vi "Is Set.vi"(8 "error in (no error)":errorcluster, 11 "Proto Type Data Base in":refnum<class "Proto Type Data Base.lvclass">) -> (0 "error out":errorcluster, 2 "Value Set":bool, 3 "Proto Type Data Base out":refnum<class "Proto Type Data Base.lvclass">)   [LabVIEW 2020, in "Protobuf RAW.lvlib" / "Proto Type Data Base.lvclass"]
uses:
  Proto Type Data Base.lvclass
  Proto Type Data Base.lvclass/Proto Type Data Base.ctl
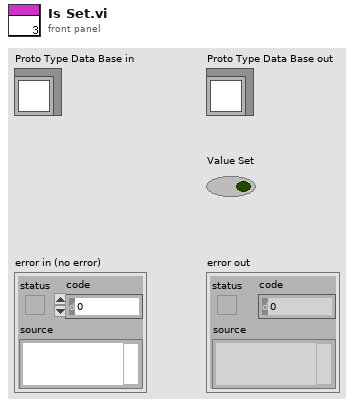
[diagram p1: front panel]
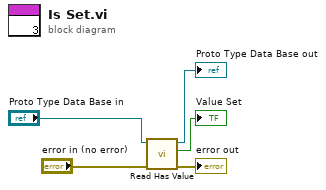
[diagram p0: block diagram]
diagram:
  n1 = call "Read Has Value.vi"("error in (no error)"="error in (no error)", "Proto Type Common in"="Proto Type Data Base in") -> ("error out"=→"error out":errorcluster, "Value Set"=→"Value Set":bool, "Proto Type Common out"=→"Proto Type Data Base out":refnum<class "Proto Type Data Base.lvclass">)  [unwired: 7 in]
